vi "RSZVB Get Converter User Data Set Directory.vi"(8 "error in (no error)":errorcluster {"code" format="%.0x"}, 10 "Port (1)":i32=1, 11 "VISA resource name":refnum<visa-resource-name>) -> (0 "error out":errorcluster {"code" format="%.0x"}, 2 "Directory":string, 3 "VISA resource name out":refnum<visa-resource-name>)   [LabVIEW 2011]
doc: "This VI returns the user data directory for the Data Set power control method.\n\nNote(s): \n\n(1) Use VI rszvb_SetSenseTypeOfPortTransferModel to set the Data Set mode.\n\n(2) Use RSZVB Set Converter Data Set Type.vi to set the User Data Set type.\n\nRemote-control command(s):\nSOURce<Ch>:POWer<Pt>:CONVerter:TRANsfer:PATH?"
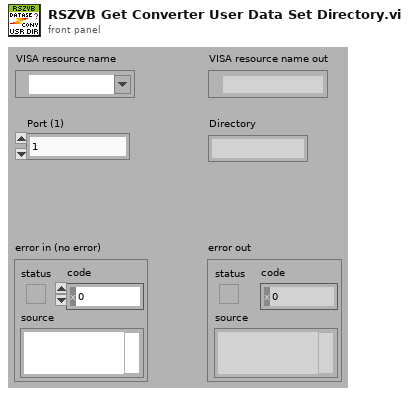
[diagram p1: front panel]
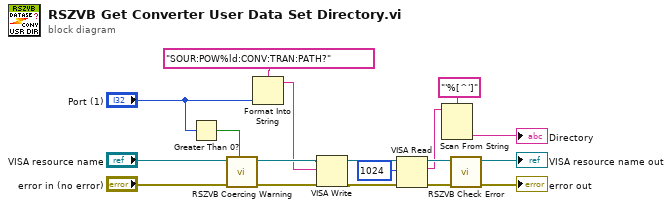
[diagram p0: block diagram]
diagram:
  n1 = Greater Than 0?(x="Port (1)") -> (x > 0?=w10:bool)
  n2 = call "RSZVB Coercing Warning.vi"("In Range?"=w10, "error in (no error)"="error in (no error)", "VISA session"="VISA resource name") -> ("error out"=w8:errorcluster, "dup VISA session"=w9:refnum<visa-resource-name>)  [unwired: 7 in]
  n3 = Format Into String(format string="SOUR:POW%ld:CONV:TRAN:PATH?", "Port (1)") -> (resulting string=w7:string)  [unwired: 2 in, 1 out]
  n4 = VISA Write(VISA resource name=w9, write buffer=w7, error in (no error)=w8) -> (VISA resource name out=w15:refnum<visa-resource-name>, error out=w14:errorcluster)  [unwired: 1 out]
  n5 = VISA Read(VISA resource name=w15, byte count=u32 1024 ("byte count (0)"), error in (no error)=w14) -> (VISA resource name out=w18:refnum<visa-resource-name>, read buffer=w12:string, error out=w17:errorcluster)  [unwired: 1 out]
  n6 = Scan From String(format string="'%[^']", input string=w12) -> (output 1=→"Directory":string)  [unwired: 3 in, 3 out]
  n7 = call "RSZVB Check Error.vi"("error in (no error)"=w17, "VISA session"=w18) -> ("error out"=→"error out":errorcluster, "dup VISA session"=→"VISA resource name out":refnum<visa-resource-name>)  [unwired: 8 in]
